vi "Test App Broadcast Nested Process Messages.vi"(8 "error in (no error)":errorcluster, 11 "Application Test In":refnum<class "Application Test.lvclass">) -> (0 "error out":errorcluster, 3 "Application Test Out":refnum<class "Application Test.lvclass">)   [LabVIEW 2020, in "Application Test.lvclass"]
uses:
  Application Test.lvclass
  C:/Program Files (x86)/National Instruments/LabVIEW 2020/vi.lib/Asteme/LUnit/Test Case.lvclass
  Mock Process/Mock Process.lvclass
  C:/Users/anton/Documents/GitHub/Triarc-Framework/source/Framework/Process/Process.lvclass
  Framework/Application/Application.lvclass
  Framework/Process/Process.lvclass/Process.ctl
  Framework/Application/Application.lvclass/Application.ctl
  <vilib>/Asteme/LUnit/Test Case.lvclass/Test Case.ctl
  <vilib>/Asteme/LUnit/LUnit Assertion Result.lvclass/LUnit Assertion Result.ctl
  Framework/Application/Private/Add Process to Map.vi
  Framework/Application/Private/Start Idle Processes if Running.vi
  Framework/Process/Protected/Messaging/Enqueue Message.vi
  Framework/Process/Public/Lifecycle/Get Lifecycle State.vi
  Framework/Process/Protected/SubVIs/Set Context.vi
  Framework/Process/Private/SubVIs/Wait for finish.vi
  Framework/Process/Private/SubVIs/Set Lifecycle State.vi
  <vilib>/Asteme/Triarc Framework/Broadcast Event Helpers/Execution timer.vi
  <vilib>/Asteme/LUnit/Palette/Pass.vi
  <vilib>/Asteme/LUnit/Palette/Fail.vi
  <vilib>/Asteme/LUnit/Variant to string.vi
  <vilib>/Asteme/LUnit/Set Assertion Type.vi
  <vilib>/Utility/error.llb/Clear Errors.vi
  Framework/Process/Public/Lifecycle/Leave Process Loop.vi
  <vilib>/Asteme/LUnit/Add test result.vi
  <vilib>/Asteme/LUnit/LUnit Write Passed.vi
  <vilib>/Asteme/LUnit/LUnit Get Test Case.vi
  <vilib>/Asteme/LUnit/Assertion Result/LUnit Get Test Name.vi
  <vilib>/Asteme/LUnit/LUnit Write Message.vi
  <vilib>/Asteme/LUnit/LUnit Write Description.vi
  <vilib>/Asteme/LUnit/LUnit Write Assertion Type.vi
  <vilib>/Asteme/LUnit/Read Test Case Name.vi
  <vilib>/Utility/error.llb/Error Cluster From Error Code.vi
  Framework/Application/Private/Throw Error If Process Already in App.vi
  Framework/Application/Private/Update Context for Owned Processes.vi
  Framework/Application/Protected/Get Broadcast Events Recursively.vi
  <vilib>/Asteme/Triarc Framework/Broadcast Event Helpers/Dequeue Broadcast Message.vi
  <vilib>/Utility/Data Type/Get Type Information.vi
  <vilib>/Utility/LVClass/Get LV Class Name.vi
  <vilib>/Asteme/LUnit/LUnit Assertion Result.lvclass
  Framework/Process/Process.lvclass
  <vilib>/Asteme/LUnit/Test Case.lvclass
  Framework/Broadcast Event Helpers/Broadcast Event Helpers.lvlib
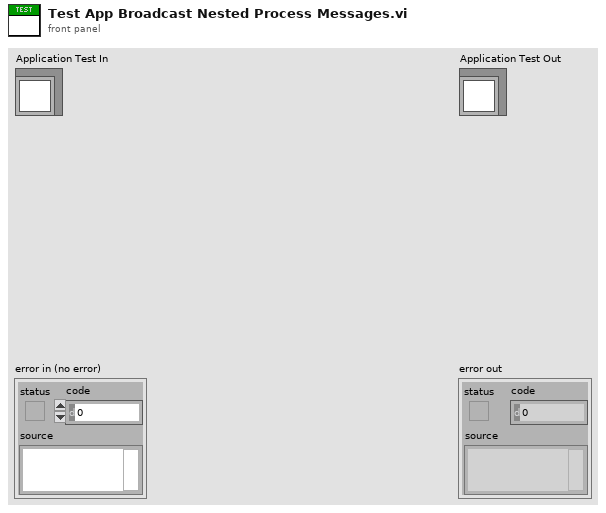
[diagram p1: front panel]
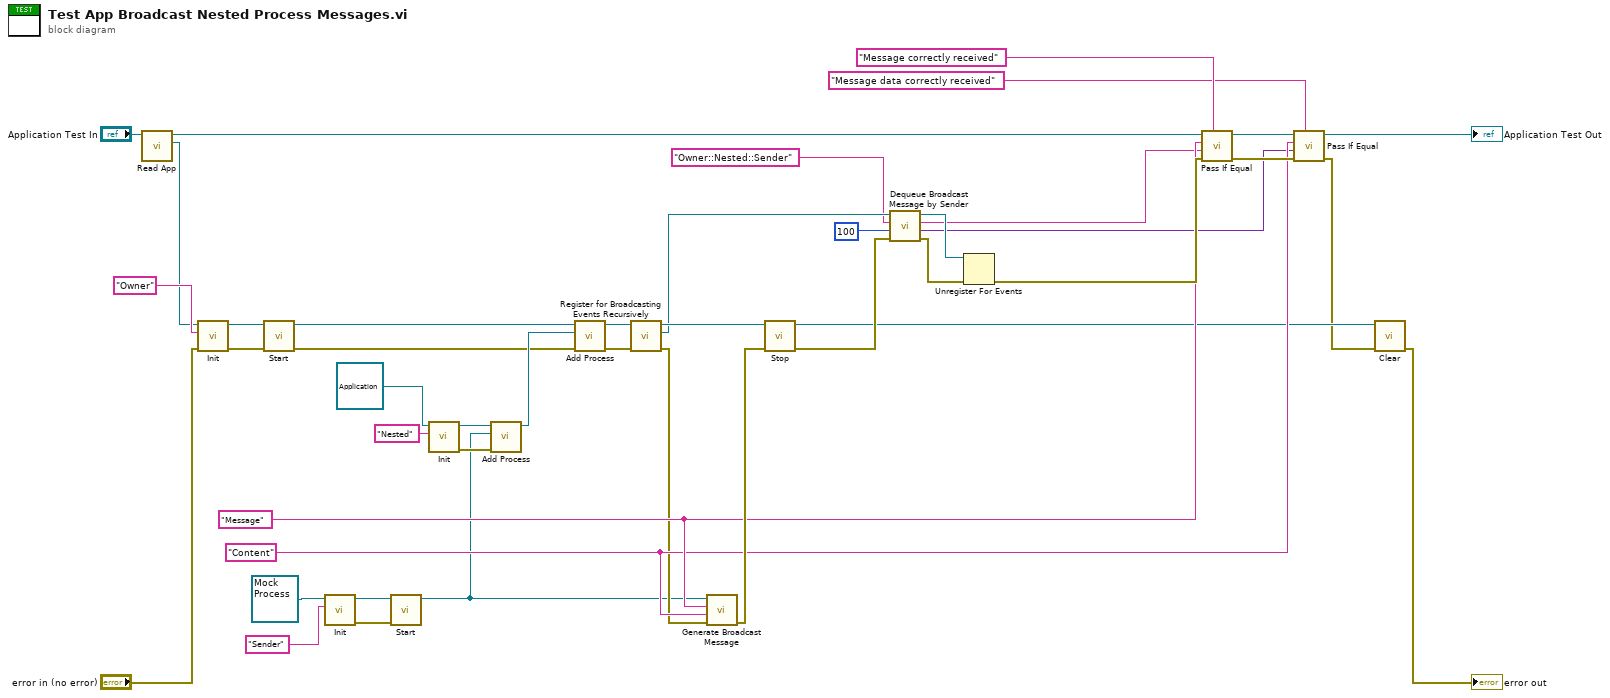
[diagram p0: block diagram]
diagram:
  w21 = "Content" ("Message")
  w22 = "Message" ("Message")
  n1 = call "Read App.vi"("Application Test In"="Application Test In") -> ("App out"=w25:refnum<class "Application.lvclass">, "Application Test Out"=w26:refnum<class "Application Test.lvclass">)  [unwired: 8 in, 1 out]
  n2 = call-dynamic "Init.vi"("error in (no error)"="error in (no error)", "Name"="Owner" ("Message"), "Process In"=w25) -> ("error out"=w42:errorcluster, "Process Out"=w43:refnum<class "Application.lvclass">)  [unwired: 7 in]
  n3 = call "Start.vi"("error in (no error)"=w42, "Process In"=w43) -> ("error out"=w2:errorcluster, "Process Out"=w39:refnum<class "Application.lvclass">)  [unwired: 7 in, 1 out]
  n4 = call-dynamic "Init.vi"("Name"="Sender" ("Message"), "Mock Process In"=refnum<class "Mock Process.lvclass"> refnum ("Mock Process.lvclass")) -> ("error out"=w29:errorcluster, "Mock Process Out"=w28:refnum<class "Mock Process.lvclass">)  [unwired: 8 in]
  n5 = call "Start.vi"("error in (no error)"=w29, "Process In"=w28) -> ("Process Out"=w5:refnum<class "Mock Process.lvclass">)  [unwired: 7 in, 2 out]
  n6 = call-dynamic "Init.vi"("Name"="Nested", "Process In"=refnum<class "Application.lvclass"> refnum ("Process Out")) -> ("error out"=w8:errorcluster, "Process Out"=w7:refnum<class "Application.lvclass">)  [unwired: 8 in]
  n7 = call "Add Process.vi"("error in (no error)"=w8, "Process"=w5, "Rig In"=w7) -> ("Rig Out"=w4:refnum<class "Application.lvclass">)  [unwired: 7 in, 1 out]
  n8 = call "Add Process.vi"("error in (no error)"=w2, "Process"=w4, "Rig In"=w39) -> ("error out"=w15:errorcluster, "Rig Out"=w16:refnum<class "Application.lvclass">)  [unwired: 7 in]
  n9 = call "Register for Broadcasting Events Recursively.vi"("error in (no error)"=w15, "Application In"=w16) -> ("error out"=w13:errorcluster, "Event Registration Refnum Out"=w12:refnum<event-registration>, "Application Out"=w14:refnum<class "Application.lvclass">)  [unwired: 7 in]
  n10 = call "Generate Broadcast Message.vi"("error in (no error)"=w13, "Message Data"=w21, "Message"=w22, "Mock Process In"=w5) -> ("error out"=w24:errorcluster)  [unwired: 6 in, 1 out]
  n11 = call "Stop.vi"("error in (no error)"=w24, "Process In"=w14) -> ("error out"=w41:errorcluster, "Process Out"=w11:refnum<class "Application.lvclass">)  [unwired: 7 in, 1 out]
  n12 = call "Dequeue Broadcast Message by Sender.vi"("error in (no error)"=w41, "Timeout (-1)"=100, "Sender"="Owner::Nested::Sender" ("Message"), "Event Registration Refnum"=w12) -> ("error out"=w17:errorcluster, "Message Data"=w19:variant, "Message"=w20:string, "Event Registration Refnum Out"=w38:refnum<event-registration>)  [unwired: 3 in, 1 out]
  n13 = Unregister For Events(event registration refnum=w38, error in=w17) -> (error out=w34:errorcluster)
  n14 = call <vilib>:"Pass If Equal.vi"("Description"="Message correctly received", "error in (no error)"=w34, "Actual"=w20, "Expected"=w22, "Test Case In"=w26) -> ("error out"=w35:errorcluster, "Test Case Out"=w36:refnum<class "Application Test.lvclass">)  [unwired: 5 in]
  n15 = call <vilib>:"Pass If Equal.vi"("Description"="Message data correctly received", "error in (no error)"=w35, "Actual"=w19, "Expected"=w21, "Test Case In"=w36) -> ("error out"=w10:errorcluster, "Test Case Out"=→"Application Test Out":refnum<class "Application Test.lvclass">)  [unwired: 5 in]
  n16 = call-dynamic "Clear.vi"("error in (no error)"=w10, "Application In"=w11) -> ("error out"=→"error out":errorcluster)  [unwired: 9 in]
